vi "Check ESTOP.vi"(8 "error in":errorcluster) -> (0 "error out":errorcluster)   [LabVIEW 2011]
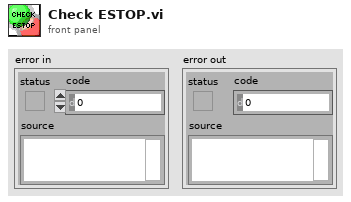
[diagram p1: front panel]
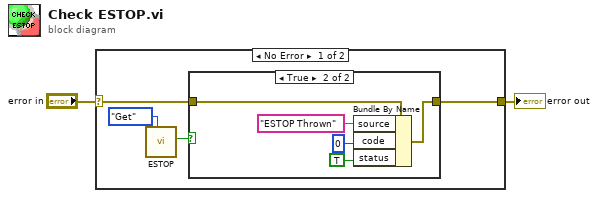
[diagram p0: block diagram]
diagram:
  n1 = case shown="No Error" "error in" {
    selector: "error in" -> [w4 w13]
    tunnel: [w3 w13] -> w1
    frame No Error {
      n2 = call "ESTOP.vi"("Get/Set"=enum16{"Get", "Set"}."Get") -> ("Value Out"=w5:bool)  [unwired: 10 in]
      n3 = case shown="True" w5 {
        tunnel: w4 -> [w7 w12]
        tunnel: [w7 w8] -> w3
        frame False {
        }
        frame True {
          n4 = Bundle By Name(cluster=w12, "source"="ESTOP Thrown", "code"=0, "status"=TRUE) -> (w8:errorcluster)
        }
      }
    }
    frame Error {
    }
  }
  "error out" <- w1
